vi "Login.vi"() -> ()   [LabVIEW 2023]
panel:
  in  "Tab Control":enum32{"Page 1", "Page 2"}(tab)
  in  "Refresh Button":bool
  in  "User":string
  in  "Password":string
  out "Answer":dbl
  in  "Numeric 2":dbl
  in  "Numeric":dbl
  in  "Stop Button":bool
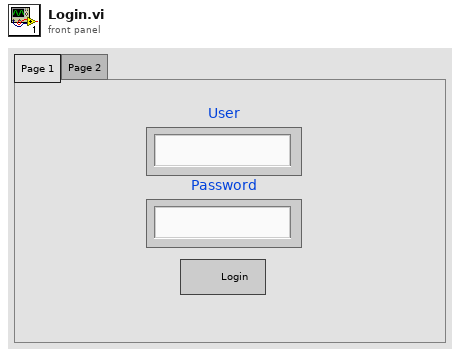
[diagram p1: front panel]
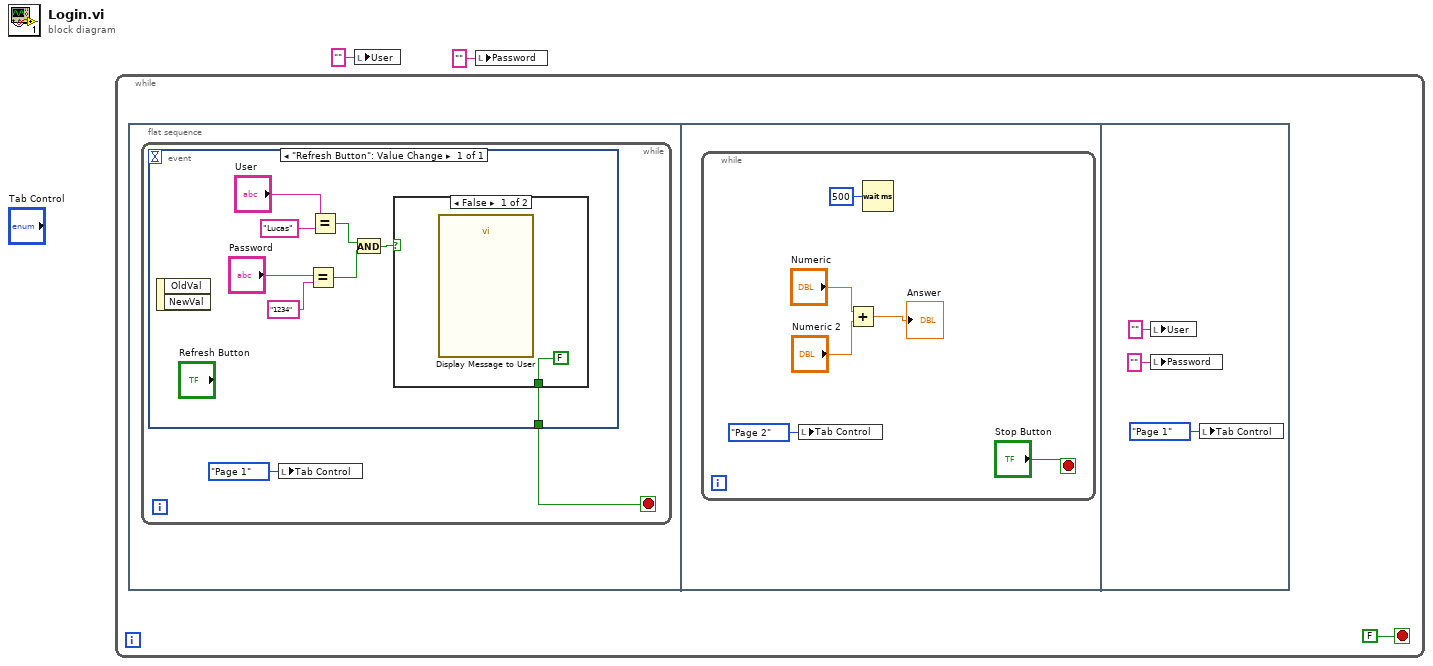
[diagram p0: block diagram]
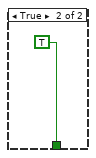
[diagram p2: hidden frame]
diagram:
  n1 = while {
    stop <- FALSE stop-if-true
    n2 = flat-sequence {
      frame #0 {
        n3 = while {
          stop <- w5 stop-if-true
          n4 = event shown="[0] \"Refresh Button\": Value Change" {
            selector: _ -> [_]
            dyn-events: _ -> [_]
            timeout: _ -> [_]
            tunnel: [w6] -> w5
            event "Refresh Button": Value Change {
              n5 = event-data() -> ()  [unwired: 1 in, 2 out]
              n6 = Equal?(x="Password", y="1234" ("x")) -> (x = y?=w8:bool)
              n7 = Equal?(x="User", y="Lucas") -> (x = y?=w9:bool)
              n8 = And(x=w9, y=w8) -> (x .and. y?=w7:bool)
              n9 = case shown="False" w7 {
                tunnel: [FALSE TRUE] -> w6
                frame False {
                  n10 = call "Display Message to User"() -> ()  [unwired: 10 in, 2 out]
                }
                frame True {
                }
              }
            }
          }
          n11 = local write "Tab Control"(enum32{"Page 1", "Page 2"}."Page 1" ("Tab Control")) -> ()
        }
      }
      frame #1 {
        n12 = while {
          stop <- "Stop Button" stop-if-true
          n13 = local write "Tab Control"(enum32{"Page 1", "Page 2"}."Page 2" ("Tab Control")) -> ()
          n14 = Add(x="Numeric", y="Numeric 2") -> (x+y=→"Answer":dbl)
          n15 = Wait (ms)(milliseconds to wait=u32 500) -> ()  [unwired: 1 out]
        }
      }
      frame #2 {
        n16 = local write "User"("" ("User")) -> ()
        n17 = local write "Password"("" ("Password")) -> ()
        n18 = local write "Tab Control"(enum32{"Page 1", "Page 2"}."Page 1" ("Tab Control")) -> ()
      }
    }
  }
  n19 = local write "User"("" ("User")) -> ()
  n20 = local write "Password"("" ("Password")) -> ()
